vi "STD浊度_获取温度和测量值.vi"(8 "error in (no error)":errorcluster caption="错误输入（无错误）", 11 "MB session in":refnum<class "MB_Master.lvclass">) -> (0 "error out":errorcluster caption="错误输出", 2 "STD浊度":cluster{"温度测量值":sgl, "浊度测量值":sgl, "信号值":sgl}, 3 "MB session out":refnum<class "MB_Master.lvclass">)   [LabVIEW 2016, in "斯坦道多参数.lvlib"]
uses:
  <vilib>/Plasmionique/MB Master/MB_Master/MB_Master.lvclass
  <vilib>/Plasmionique/MB Master/MB Master.lvlib
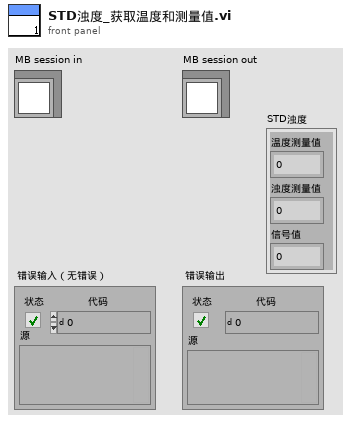
[diagram p1: front panel]
types:
  T1 = cluster{"pH":u32, "DO":u32, "Cond":u32, "Turb":u32, "叶绿素a":u32, "藻密度":u32, "ORP":u32, "COD":u32, "氯化物":u32, "氨氮":u32, "水中油":u32}
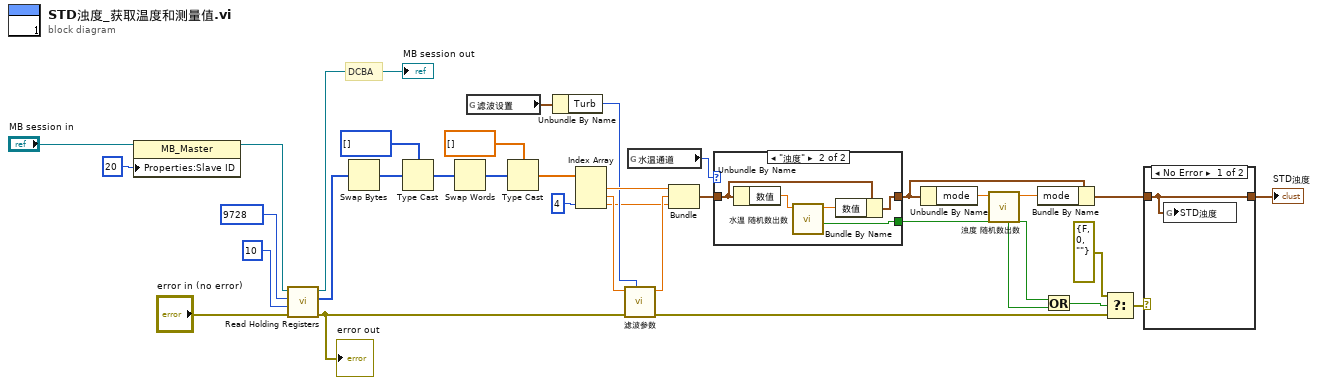
[diagram p0: block diagram]
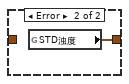
[diagram p3: hidden frame]
diagram:
  # "DCBA"
  n1 = property class="MB_Master"(reference="MB session in", "Properties:Slave ID"=u16 20 ("y")) -> (reference out=w27:refnum<class "MB_Master.lvclass">)  [unwired: 1 in, 1 out]
  n2 = call <vilib>:"Read Holding Registers.vi"("error in (no error)"="error in (no error)", "quantity"=u16 10, "starting address"=u16 9728, "MB session in"=w27) -> ("error out"=w16:errorcluster, "Registers"=w25:u16[], "MB session out"=→"MB session out":refnum<class "MB_Master.lvclass">)  [unwired: 5 in]
  "error out" <- w16
  n3 = Swap Bytes(anything=w25) -> (byte swapped=w24:u16[])
  n4 = Type Cast(type=u32[] [] ("数组 2"), x=w24) -> (*(type *) &x=w31:u32[])
  n5 = Swap Words(1:w31) -> (0:w33:u32[])
  n6 = global read "断电保存变量.vi" "滤波设置"() -> (w18:T1)
  n7 = Type Cast(type=sgl[] [] ("数组 2"), x=w33) -> (*(type *) &x=w29:sgl[])
  n8 = Unbundle By Name(w18) -> ("Turb"=w17:u32)
  n9 = Index Array(array=w29, index #3=4 ("索引")) -> (element #1=w23:sgl, element #2=w20:sgl, element #3=w14:sgl)  [unwired: 2 in]
  n10 = call "滤波参数.vi"("滤波次数"=w17, "error in (no error)"=w16, "x"=w20) -> ("error out"=w3:errorcluster, "mode"=w19:dbl)  [unwired: 7 in]
  n11 = global read "断电保存变量.vi" "水温通道"() -> (w11:enum16{"pH", "DO", "浊度", "电导率", "叶绿素a", "藻密度"})
  n12 = Bundle("数值"=w23, "mode"=w19, "数值"=w14) -> (w10:cluster{"数值":sgl, "mode":dbl, "数值":sgl})  [unwired: 1 in]
  n13 = case shown="\"浊度\"" w11 {
    tunnel: w10 -> [w36 w40]
    tunnel: [w36 w38] -> w9
    tunnel: [_ w37] -> w5
    frame Default {
    }
    frame "浊度" {
      n14 = Unbundle By Name(w40) -> ("数值"=w41:sgl)
      n15 = call "水温 随机数出数.vi"("原始值"=w41) -> ("取值输出"=w39:dbl, "x .and. y?"=w37:bool)  [unwired: 6 in, 1 out]
      n16 = Bundle By Name(cluster=w40, "数值"=w39) -> (w38:cluster{"数值":sgl, "mode":dbl, "数值":sgl})
    }
  }
  n17 = Unbundle By Name(w9) -> ("mode"=w13:dbl)
  n18 = call "浊度 随机数出数.vi"("原始值"=w13) -> ("取值输出"=w12:dbl, "x .and. y?"=w6:bool)  [unwired: 6 in, 1 out]
  n19 = Bundle By Name(cluster=w9, "mode"=w12) -> (w8:cluster{"数值":sgl, "mode":dbl, "数值":sgl})
  n20 = Or(x=w5, y=w6) -> (x .or. y?=w4:bool)
  n21 = Select(t=errorcluster {"status"=FALSE, "code"=0, "source"=""}, s=w4, f=w3) -> (s? t:f=w2:errorcluster)
  n22 = case shown="No Error" w2 {
    tunnel: w8 -> [w42 _]
    tunnel: [w42 w43] -> w7
    frame No Error {
      n23 = global write "禹山过程全局变量.vi" "STD浊度"(w42) -> ()
    }
    frame Error {
      n24 = global read "禹山过程全局变量.vi" "STD浊度"() -> (w43:cluster{"温度测量值":sgl, "浊度测量值":sgl, "信号值":sgl})
    }
  }
  "STD浊度" <- w7
